vi "MU error coding.vi"(8 "error in (no error)":errorcluster, 11 "function return in":u32) -> (0 "error out":errorcluster)   [LabVIEW 2022 SP3, in "MU_3SL_interface.lvlib"]
uses:
  MU_3SL_interface.lvlib
  enums/MU_Error.ctl
panel:
  in  "MU_ErrorEnum":T1
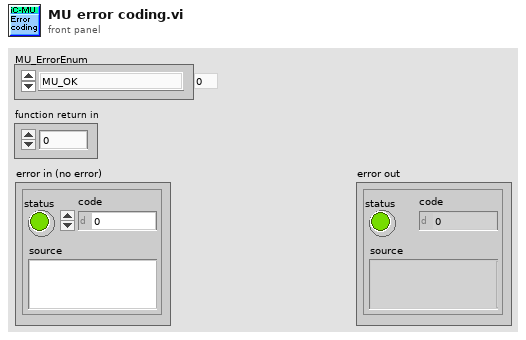
[diagram p1: front panel]
types:
  T1 = typedef "MU_3SL_interface.lvlib/MU_Error.ctl" = enum32{"MU_OK", "MU_INVALID_HANDLE", "MU_INTERFACEDRIVER_NOT_FOUND", "MU_INTERFACE_NOT_FOUND", "MU_INVALID_INTERFACE", "MU_NO_INTERFACE_SELECTED", "MU_INVALID_PARAMETER", "MU_INVALID_ADDRESS", "MU_INVALID_VALUE", "MU_USB_ERROR", "MU_FILE_NOT_FOUND", "MU_INVALID_FILE", "MU_SPI_ERROR", "MU_SPI_DISMISS", "MU_SPI_FAIL", "MU_SPI_BUSY_TIMEOUT", "MU_VERIFY_FAILED", "MU_MASTERCOMM_FAILED", "MU_BISSCOMM_FAILED", "MU_INVALID_BISSMASTER", "MU_USB_HIGHSPEED_WARNING", "MU_FAST_ROTATION", "MU_SLOW_ROTATION", "MU_FILE_ACCESS_DENIED", "MU_READPARAM_SSI", "MU_SSIRING_ERROR", "MU_SEMI_ROTATION", "MU_BISS_REGERROR", "MU_INTERNAL_CALIB_ERROR", "MU_INVALID_CONFIGURATION", "MU_CALIBRATION_FAILED", "MU_ACQUISITION_FAILED", "MU_GAIN_LIMIT", "MU_OFFSET_LIMIT", "MU_PHASE_LIMIT", "MU_BAD_CAL_DATA", "MU_I2C_COMM_FAILED", "MU_USB_DATA_LOSS", "MU_MT_SYNC_FAILED", "MU_UNKNOWN_ERROR", "MU_UNKNOWN_REVISION", "MU_UNSUPPORTED_REVISION", "MU_UNKNOWN_PARAMETER", "MU_PARAMETER_NOT_IN_REVISION", "MU_REVISION_NOT_SET", "MU_UNSUPPORTED_CHIP", "MU_CONTRADICTORY_REVISIONS", "MU_FRAME_RATE_NOT_SUPPORTED", "MU_CLOCK_FREQUENCY_NOT_SUPPORTED", "MU_FRAME_CYCLE_TIME_TO_SHORT", "MU_NO_BISS_PROFILE_ID", "MU_ADAPTER_FIRMWARE_INCOMPATIBLE"}
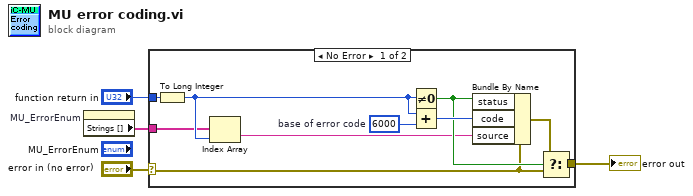
[diagram p0: block diagram]
diagram:
  n1 = property on="MU_ErrorEnum" class="Enum (strict)"() -> ("Strings []"=w1:string[])  [unwired: 2 in, 2 out]
  n2 = case shown="No Error" "error in (no error)" {
    selector: "error in (no error)" -> [w9 w15]
    tunnel: [w8 w15] -> w3
    tunnel: "function return in" -> [w13 _]
    tunnel: w1 -> [w6 _]
    frame No Error {
      w14 = 6000  # base of error code
      n3 = To Long Integer(number=w13) -> (32bit integer=w7:i32)
      n4 = Index Array(array=w6, index=w7) -> (element=w5:string)
      n5 = Not Equal To 0?(x=w7) -> (x != 0?=w11:bool)
      n6 = Add(x=w7, y=w14) -> (x+y=w12:i32)
      n7 = Bundle By Name(cluster=w9, "status"=w11, "code"=w12, "source"=w5) -> (w10:errorcluster)
      n8 = Select(t=w10, s=w11, f=w9) -> (s? t:f=w8:errorcluster)
    }
    frame Error {
    }
  }
  "error out" <- w3
